vi "Filter References.vi"(7 "Config out":refnum<class "TAF Proj Config.lvclass">, 10 "VI References in":refnum<vi>[](array[refnum]), 11 "Library References in":refnum<vi>[](array[refnum])) -> (2 "VI References out":refnum<vi>[](array[refnum]), 3 "Library References out":refnum<vi>[](array[refnum]))   [LabVIEW 2021, in "TAF Proj Document Type.lvlib" / "Project Parser.lvlib"]
uses:
  <vilib>/Wovalab/AntiDoc/Document Type/Add-ons/LabVIEW TAF Project/Project Parser/Project Parser.lvlib
  <vilib>/Wovalab/AntiDoc/Document Type/Add-ons/LabVIEW TAF Project/TAF Proj Config/TAF Proj Config.lvclass
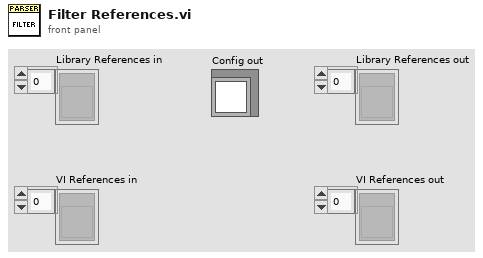
[diagram p1: front panel]
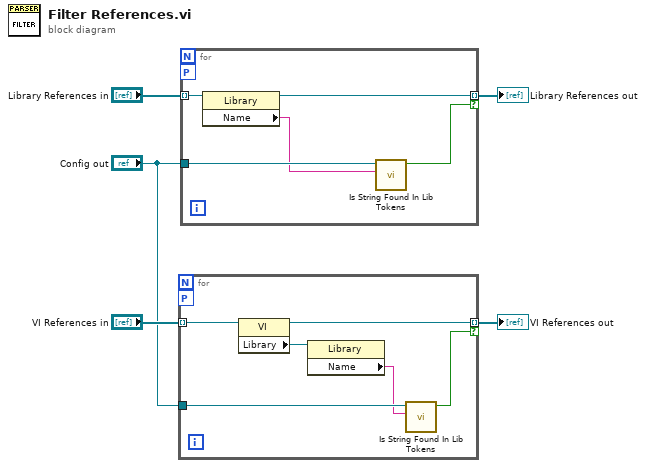
[diagram p0: block diagram]
diagram:
  n1 = for {
    tunnel: "VI References in" -> [w11] mode=indexing
    tunnel: [w10] -> w3 mode=indexing if=w7
    workers-P: _ -> [_]
    tunnel: "Config out" -> [w8]
    n2 = property class="VI"(reference=w11) -> (reference out=w10:refnum<vi>, "Library"=w9:refnum<vi>)  [unwired: 1 in, 1 out]
    n3 = property class="Library"(reference=w9) -> ("Name"=w6:string)  [unwired: 1 in, 2 out]
    n4 = call <vilib>:"Is String Found In Lib Tokens.vi"("String"=w6, "Config"=w8) -> ("Not Found?"=w7:bool)  [unwired: 9 in]
  }
  "VI References out" <- w3
  n5 = for {
    tunnel: "Library References in" -> [w16] mode=indexing
    tunnel: [w15] -> w4 mode=indexing if=w14
    workers-P: _ -> [_]
    tunnel: "Config out" -> [w13]
    n6 = property class="Library"(reference=w16) -> (reference out=w15:refnum<vi>, "Name"=w12:string)  [unwired: 1 in, 1 out]
    n7 = call <vilib>:"Is String Found In Lib Tokens.vi"("String"=w12, "Config"=w13) -> ("Not Found?"=w14:bool)  [unwired: 9 in]
  }
  "Library References out" <- w4
